vi "pmu_Get Elements To Read.vi"(0 "timestamps":dbl[][](array[numeric]), 1 "min tfinal":timestamp, 2 "reset? (F)":bool, 5 "max t0 index":i32, 7 "performance class":enum8{"M Class", "P Class"}(ring), 9 "reporting time":timestamp, 11 "reporting rate":dbl, 12 "window length":i32, 13 "initial samples to read":u32) -> (4 "elements to read":u32)   [LabVIEW 2013, in "NI_EP_PMU.lvlib"]
uses:
  <vilib>/addons/Electrical Power/PMU/NI_EP_PMU.lvlib
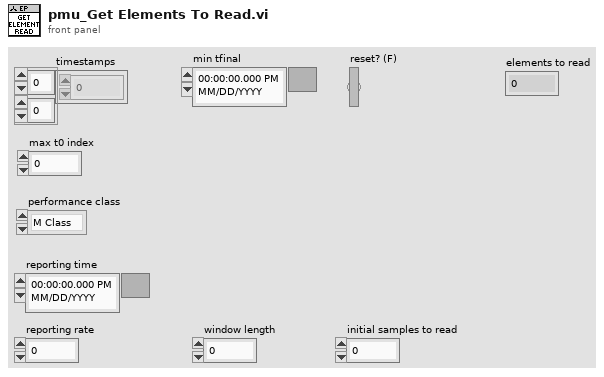
[diagram p1: front panel]
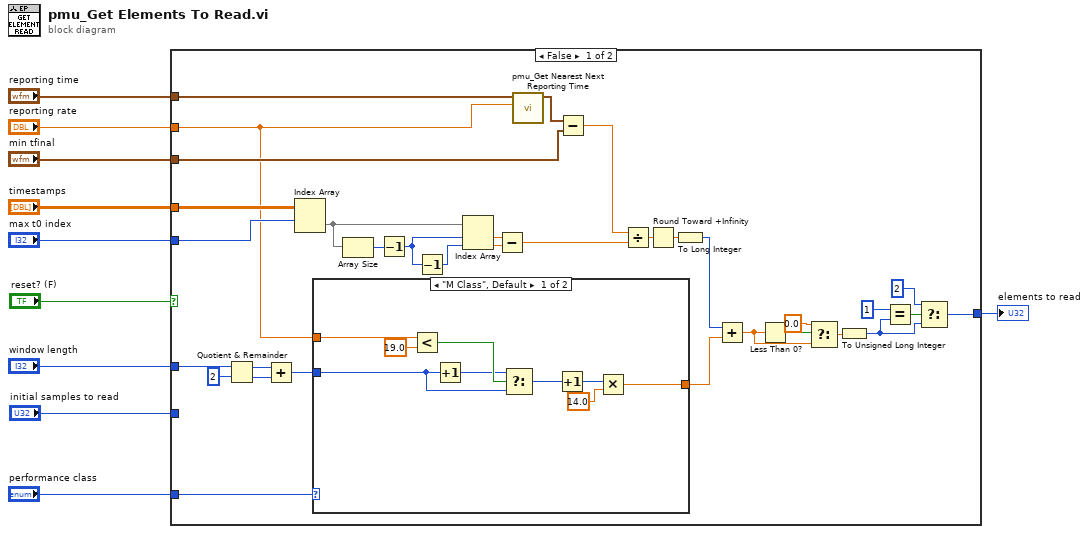
[diagram p0: block diagram]
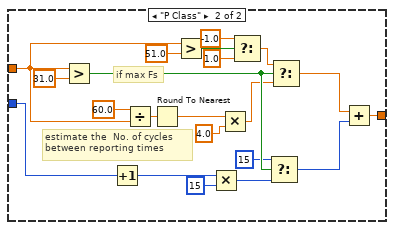
[diagram p2: hidden frame]
diagram:
  n1 = case shown="False" "reset? (F)" {
    tunnel: "reporting rate" -> [w18 _]
    tunnel: "max t0 index" -> [w43 _]
    tunnel: "timestamps" -> [w42 _]
    tunnel: "min tfinal" -> [w41 _]
    tunnel: "window length" -> [w14 _]
    tunnel: "reporting time" -> [w40 _]
    tunnel: [w31 w74] -> w4
    tunnel: "initial samples to read" -> [_ w74]
    tunnel: "performance class" -> [w16 _]
    frame False {
      n2 = Quotient & Remainder(x=w14, y=2) -> (x-y*floor(x/y)=w12:i32, floor(x/y)=w11:i32)
      n3 = Add(x=w12, y=w11) -> (x+y=w13:i32)
      n4 = Index Array(array=w42, index (row)=w43) -> (element=w37:dbl[])  [unwired: 1 in]
      n5 = case shown="\"M Class\", Default" w16 {
        tunnel: w18 -> [w50 w58]
        tunnel: [w48 w65] -> w17
        tunnel: w13 -> [w44 w61]
        frame "M Class", Default {
          n6 = Less?(x=w50, y=19.0) -> (x < y?=w46:bool)
          n7 = Increment(x=w44) -> (x+1=w45:i32)
          n8 = Select(t=w45, s=w46, f=w44) -> (s? t:f=w47:i32)
          n9 = Increment(x=w47) -> (x+1=w52:i32)
          n10 = Multiply(x=w52, y=14.0) -> (x*y=w48:dbl)
        }
        frame "P Class" {
          # "estimate the  No. of cycles \nbetween reporting times"
          # "if max Fs"
          n11 = Greater?(x=w58, y=31.0) -> (0:w68:bool)
          n12 = Increment(x=w61) -> (x+1=w60:i32)
          n13 = Divide(x=60.0 ("y"), y=w58) -> (x/y=w71:dbl)
          n14 = Round To Nearest(number=w71) -> (nearest integer value=w64:dbl)
          n15 = Greater?(x=w58, y=51.0) -> (0:w56:bool)
          n16 = Multiply(x=w60, y=u32 15) -> (x*y=w63:u32)
          n17 = Multiply(x=w64, y=4.0) -> (x*y=w67:dbl)
          n18 = Select(t=-1.0, s=w56, f=1.0 ("t")) -> (s? t:f=w57:dbl)
          n19 = Select(t=u32 15 ("y"), s=w68, f=w63) -> (s? t:f=w73:u32)
          n20 = Select(t=w57, s=w68, f=w67) -> (s? t:f=w53:dbl)
          n21 = Add(x=w53, y=w73) -> (x+y=w65:dbl)
        }
      }
      n22 = Array Size(array=w37) -> (size(s)=w36:i32)
      n23 = Decrement(x=w36) -> (x-1=w34:i32)
      n24 = Decrement(x=w34) -> (x-1=w35:i32)
      n25 = Index Array(array=w37, index #1=w34, index #2=w35) -> (element #1=w33:dbl, element #2=w32:dbl)
      n26 = Subtract(x=w33, y=w32) -> (x-y=w30:dbl)
      n27 = call <vilib>:"pmu_Get Nearest Next Reporting Time.vi"("reporting rate"=w18, "time in"=w40) -> ("reporting time"=w39:timestamp)  [unwired: 8 in, 1 out]
      n28 = Subtract(x=w39, y=w41) -> (x-y=w38:dbl)
      n29 = Divide(x=w38, y=w30) -> (x/y=w23:dbl)
      n30 = Round Toward +Infinity(x=w23) -> (ceil(x): smallest int >= x=w24:dbl)
      n31 = To Long Integer(number=w24) -> (32bit integer=w25:i32)
      n32 = Add(x=w25, y=w17) -> (x+y=w28:dbl)
      n33 = Less Than 0?(x=w28) -> (x < 0?=w27:bool)
      n34 = Select(t=0.0, s=w27, f=w28) -> (s? t:f=w29:dbl)
      n35 = To Unsigned Long Integer(number=w29) -> (unsigned 32bit integer=w19:u32)
      n36 = Equal?(x=u32 1, y=w19) -> (x = y?=w21:bool)
      n37 = Select(t=u32 2 ("x"), s=w21, f=w19) -> (s? t:f=w31:u32)
    }
    frame True {
    }
  }
  "elements to read" <- w4
